vi "Setup UI.vi"(8 "error in (no error)":errorcluster, 10 "Set UI to input? (F)":bool, 11 "Magna Power Scan in":refnum<class "Magna Power Scan.lvclass">) -> (0 "error out":errorcluster, 3 "Magna Power Scan out":refnum<class "Magna Power Scan.lvclass">)   [LabVIEW 2012, in "Magna Power Scan.lvclass"]
doc: "Scanner::Setup is a constructor that has no parameters and faces the user. The Factory calls this VI to let the user configure this Scanner. It is dynamically dispatched in order to let the user choose the type as well as the options of the scanner."
uses:
  Magna Power Scan.lvclass
  Magna Power Scan.lvclass/Magna Power Scan.ctl
  Instruments/Magna-Power Power Supply/Magna Power.lvclass
  Instruments/Magna-Power Power Supply/Magna Power Constants.vi
  <vilib>/gmath/NI_Gmath.lvlib
panel:
  out "Positive?":bool
  in  "Go to first\ncoordinate (roughly)":bool
  in  "Sweep rate (T/s)":dbl
  in  "Voltage Limit":dbl=2255.0
  # "Magna Power Continuous Setup"
  # "A positive field corresponds to a north pole located on the right when looking straight on at magnet"
  # "Usually set to 2255 V"
  # "(Button will stay\ngreen when pressed)"
  # "Max field ~ 1.36 T\nAlways enter positive field values.\n\nMay behave strangely for fields below 0.05 T,\nbut a \"Return to\" value of 0 is valid."
  # "If you want to do multiple scans, you must check the \"Return to\" box and enter the first point of your scan."
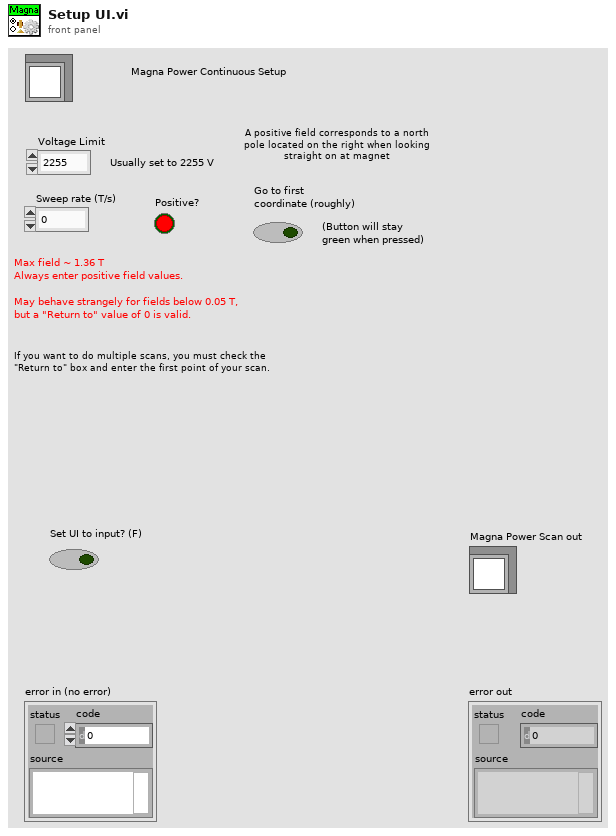
[diagram p1: front panel]
types:
  T1 = typedef "Scanner.lvclass/Range.ctl" = cluster{"xi":dbl, "xf":dbl, "dx":dbl, "Return to...?":bool, "Return to":dbl}
  T2 = cluster{"Magna Current":dbl[], "Magnetic Field":dbl[], "Fluke Voltage":dbl[]}
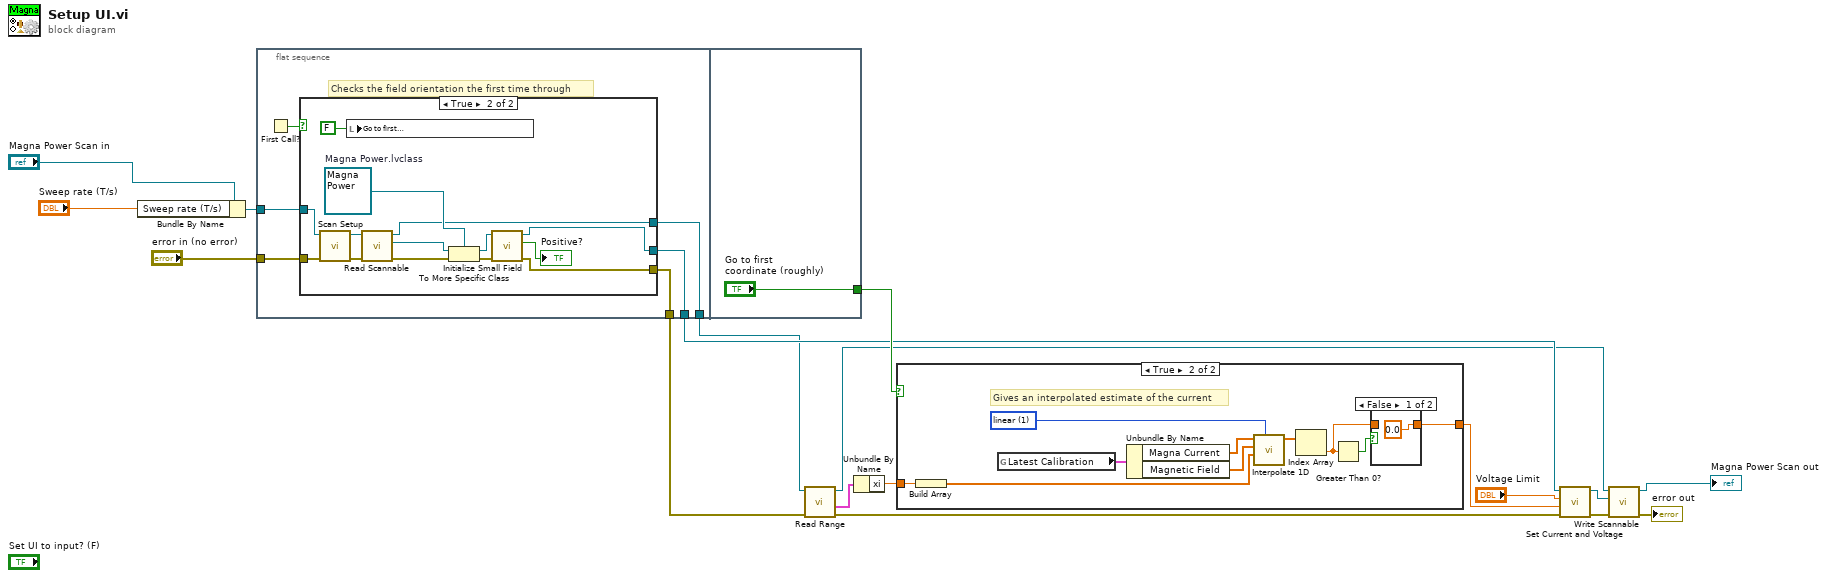
[diagram p0: block diagram]
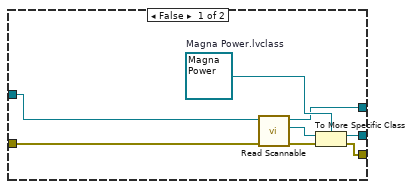
[diagram p2: hidden frame]
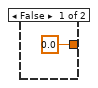
[diagram p3: hidden frame]
diagram:
  n1 = Bundle By Name(cluster="Magna Power Scan in", "Sweep rate (T/s)"="Sweep rate (T/s)") -> (w10:refnum<class "Magna Power Scan.lvclass">)
  n2 = flat-sequence {
    tunnel: "error in (no error)" -> [w23]
    tunnel: w10 -> [w22]
    tunnel: [w21] -> w3
    tunnel: [w20] -> w5
    tunnel: [w19] -> w9
    tunnel: ["Go to first\ncoordinate (roughly)"] -> w13
    frame #0 {
      # "Checks the field orientation the first time through"
      n3 = First Call?() -> (First Call?: T/F=w24:bool)
      n4 = case shown="True" w24 {
        tunnel: w22 -> [w31 w42]
        tunnel: w23 -> [w27 w41]
        tunnel: [w30 w36] -> w21
        tunnel: [w26 w35] -> w20
        tunnel: [w25 w33] -> w19
        frame False {
          w32 = refnum<class "Magna Power.lvclass"> refnum  # Magna Power.lvclass
          n5 = call-dynamic "Read Scannable.vi"("error in (no error)"=w27, "Scanner.lvclass in"=w31) -> ("error out"=w29:errorcluster, "Scannable.lvclass"=w28:refnum<class "Scannable.lvclass">, "Scanner.lvclass out"=w30:refnum<class "Magna Power Scan.lvclass">)  [unwired: 7 in]
          n6 = To More Specific Class(target class=w32, reference=w28, error in=w29) -> (specific class reference=w25:refnum<class "Magna Power.lvclass">, error out=w26:errorcluster)
        }
        frame True {
          w44 = refnum<class "Magna Power.lvclass"> refnum  # Magna Power.lvclass
          n7 = call-dynamic "Scan Setup.vi"("error in (no error)"=w41, "Magna Power Scan in"=w42) -> ("error out"=w39:errorcluster, "Magna Power Scan out"=w40:refnum<class "Magna Power Scan.lvclass">)  [unwired: 8 in]
          n8 = local write "Go to first\ncoordinate (roughly)"(FALSE ("Go to first coordinate (roughly)")) -> ()
          n9 = call-dynamic "Read Scannable.vi"("error in (no error)"=w39, "Scanner.lvclass in"=w40) -> ("error out"=w45:errorcluster, "Scannable.lvclass"=w43:refnum<class "Scannable.lvclass">, "Scanner.lvclass out"=w36:refnum<class "Magna Power Scan.lvclass">)  [unwired: 7 in]
          n10 = To More Specific Class(target class=w44, reference=w43, error in=w45) -> (specific class reference=w37:refnum<class "Magna Power.lvclass">, error out=w38:errorcluster)
          n11 = call "Initialize Small Field.vi"("error in (no error)"=w38, "Magna Power in"=w37) -> ("error out"=w35:errorcluster, "Positive?"=→"Positive?":bool, "Magna Power out"=w33:refnum<class "Magna Power.lvclass">)  [unwired: 7 in]
        }
      }
    }
    frame #1 {
    }
  }
  n12 = call-dynamic "Read Range.vi"("error in (no error)"=w5, "Scanner.lvclass in"=w3) -> ("error out"=w4:errorcluster, "Range"=w6:T1, "Scanner.lvclass out"=w2:refnum<class "Magna Power Scan.lvclass">)  [unwired: 4 in, 3 out]
  n13 = Unbundle By Name(w6) -> ("xi"=w1:dbl)
  n14 = case shown="True" w13 {
    tunnel: [0.0 ("Current Limit") w50] -> w12
    tunnel: w1 -> [_ w49]
    frame False {
    }
    frame True {
      w57 = 1 items=["nearest", "linear", "spline", "cubic Hermite", "Lagrange"] ("method")
      # "Gives an interpolated estimate of the current"
      n15 = Build Array(w49) -> (w56:dbl[])
      n16 = global read "Magna Power Constants.vi" "Latest Calibration"() -> (w58:T2)
      n17 = Unbundle By Name(w58) -> ("Magna Current"=w53:dbl[], "Magnetic Field"=w54:dbl[])
      n18 = call <vilib>:"Interpolate 1D.vi"("method"=w57, "xi"=w56, "X"=w54, "Y"=w53) -> ("yi"=w55:dbl[])  [unwired: 5 in, 2 out]
      n19 = Index Array(array=w55) -> (element=w51:dbl)  [unwired: 1 in]
      n20 = Greater Than 0?(x=w51) -> (x > 0?=w52:bool)
      n21 = case shown="False" w52 {
        tunnel: [0.0 ("Numeric") w60] -> w50
        tunnel: w51 -> [_ w60]
        frame False {
        }
        frame True {
        }
      }
    }
  }
  n22 = call "Set Current and Voltage.vi"("error in (no error)"=w4, "Current Limit"=w12, "Voltage Limit"="Voltage Limit", "Magna Power in"=w9) -> ("error out"=w18:errorcluster, "Magna Power out"=w17:refnum<class "Magna Power.lvclass">)  [unwired: 6 in]
  n23 = call-dynamic "Write Scannable.vi"("error in (no error)"=w18, "Scannable.lvclass"=w17, "Scanner.lvclass in"=w2) -> ("error out"=→"error out":errorcluster, "Scanner.lvclass out"=→"Magna Power Scan out":refnum<class "Magna Power Scan.lvclass">)  [unwired: 7 in]
